vi "Correlation Coefficient.vi"(10 "Y":dbl[](array[numeric]) format="%.2f", 11 "X":dbl[](array[numeric]) format="%.2f") -> (2 "r^2":dbl format="%.7g", 3 "correlation coefficient r":dbl format="%.7g")   [LabVIEW 2020, in "NI_Gmath.lvlib"]
doc: "Computes the linear correlation coefficient between input sequences <B>X</B> and <B>Y</B>."
uses:
  <vilib>/gmath/NI_Gmath.lvlib
  <vilib>/Analysis/NI_AALBase.lvlib
panel:
  # "Correlation Coefficient \n(Pearson)"
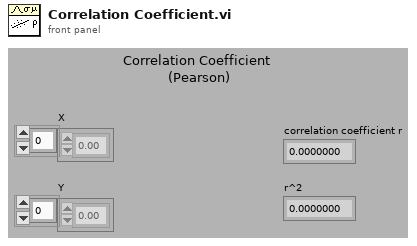
[diagram p1: front panel]
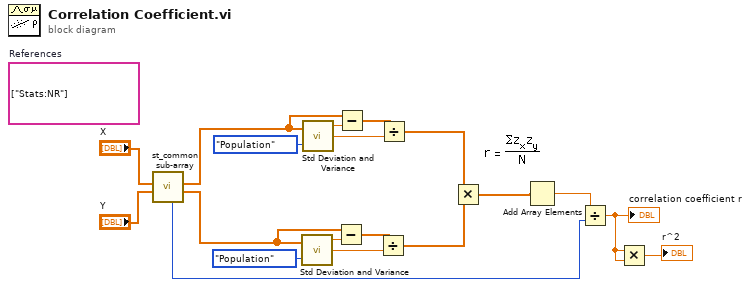
[diagram p0: block diagram]
diagram:
  (unwired) string[] ["Stats:NR"]  # References
  n1 = call <vilib>:"st_common sub-array.vi"(9:"array 1 in"="Y", 10:"array 1 in"="X") -> (1:"array 1 out"=w2:dbl[], 2:"array 1 out"=w3:dbl[], "size"=w16:i32)  [unwired: 7 in]
  n2 = call <vilib>:"Std Deviation and Variance.vi"("X"=w2, "Weighting (Sample)"=enum16{"Sample", "Population"}."Population") -> ("mean"=w4:dbl, "standard deviation"=w6:dbl)  [unwired: 1 out]
  n3 = call <vilib>:"Std Deviation and Variance.vi"("X"=w3, "Weighting (Sample)"=enum16{"Sample", "Population"}."Population") -> ("mean"=w13:dbl, "standard deviation"=w11:dbl)  [unwired: 1 out]
  n4 = Subtract(x=w2, y=w4) -> (x-y=w5:dbl[])
  n5 = Subtract(x=w3, y=w13) -> (x-y=w12:dbl[])
  n6 = Divide(x=w5, y=w6) -> (x/y=w1:dbl[])
  n7 = Divide(x=w12, y=w11) -> (x/y=w10:dbl[])
  n8 = Multiply(x=w10, y=w1) -> (x*y=w9:dbl[])
  n9 = Add Array Elements(numeric array=w9) -> (sum=w19:dbl)
  n10 = Divide(x=w19, y=w16) -> (x/y=w18:dbl)
  "correlation coefficient r" <- w18
  n11 = Multiply(x=w18, y=w18) -> (x*y=→"r^2":dbl)
